vi "TemperatureControl_AVS.vi"(0 "T target":dbl, 5 "rate (K/min)":dbl=0.001, 9 "stop":bool, 11 "wait for T":bool, 12 "heater off":bool) -> (4 "T_set = T_target":bool)   [LabVIEW 2010]
uses:
  Instrument_Setup.vi
  Data_Display_global.vi
  Instance           1 36Saved   Temperaturkontrolle_Anfahren .vi
  Programme/National Instruments/LabVIEW 8.5/instr.lib/Mischerinstr.lib/AVS-Brücke/LV Drivers for AVS/AVS47IB.LLB/AVS47IB Wait for OPC/MAV/TMO.vi
  ControlCentre/Global 1.vi
panel:
  in  "Still value (mA)":dbl=0.7
  out "R":dbl=22.359058380126953 format="%.2f"
  out "activity":bool
  in  "excitation low T":dbl=4.0
  in  "change excitation":bool
  in  "excitation high T":dbl=4.0
  in  "from T (K)":dbl=0.15
  in  "?":bool
  in  "wait after sweep":u32
  in  "T max \nstill=on":dbl=0.7
  in  "still automatic":bool
  out "i=0":bool
  in  "change rate":bool
  in  "?":bool
  out "stability (K)":dbl
  in  "wait before start":u32=30
  in  "High-T mode":bool
  in  "from T (K)":dbl=0.5
  in  "change rate\nK/min":dbl=0.015
  in  "Delay (sec) 2":i16=1 min=0 max=3600 step=1
  out "T within\ntolerance":bool
  in  "stability \ntolerance (%)":dbl=1.0
  out "SetPoint":dbl
  out "T_set":dbl
  out "Delta t (sec)":dbl format="%.4f"
  in  "Delay (sec)":i16=1 min=0 max=3600 step=1
  out "T (K)":dbl=0.00957168277075326 format="%^.3e"
  in  "sweep tolerance %":dbl=0.1
  in  "critical temperature":dbl=0.8
  out "?":bool
  out "Down-Sweep":bool
  in  "tolerance T_set=T_target %":dbl=0.1
  out "resistance":dbl format="%.2f"
  out "T(K) history 2":dbl(graph)
  out "K  2":dbl format="%.4f"
  out "T(K) history3":dbl(graph)
  out "K":dbl format="%.4f"
  # "s"
  # "s"
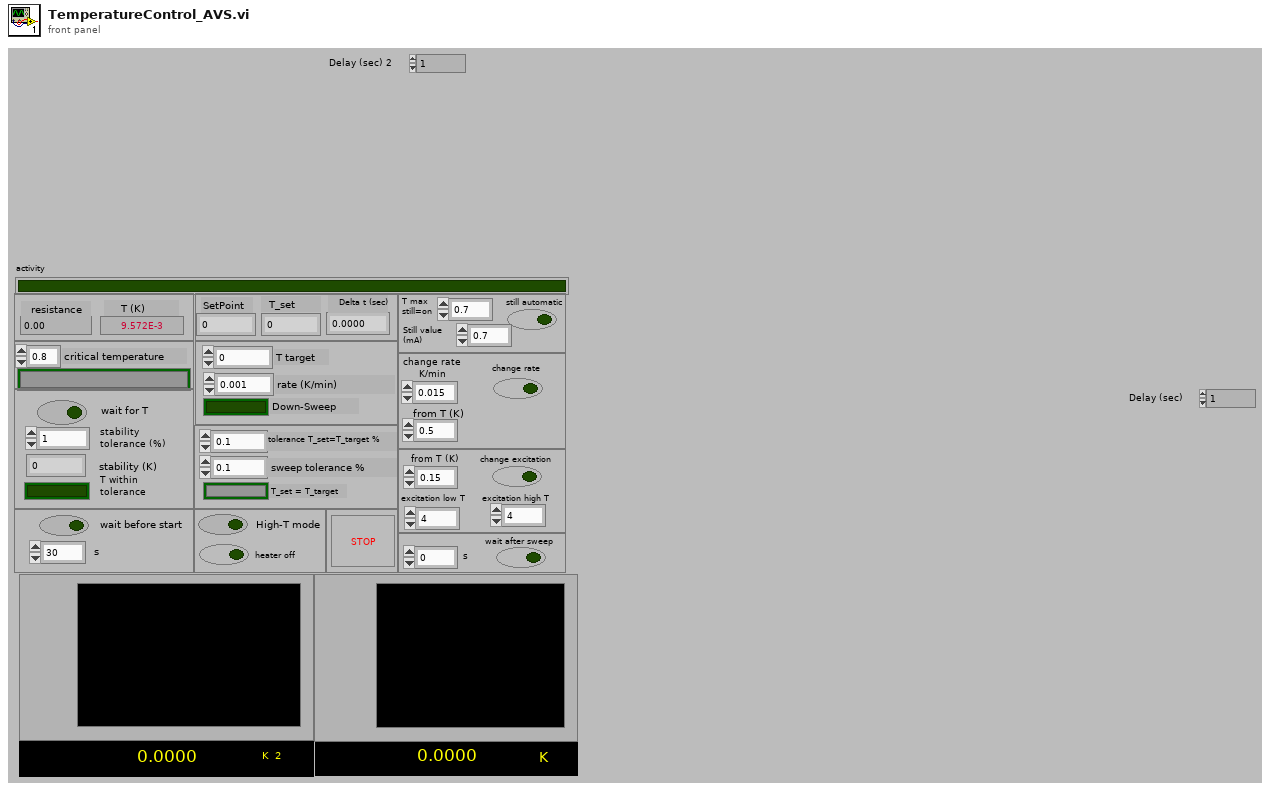
[diagram p1: front panel]
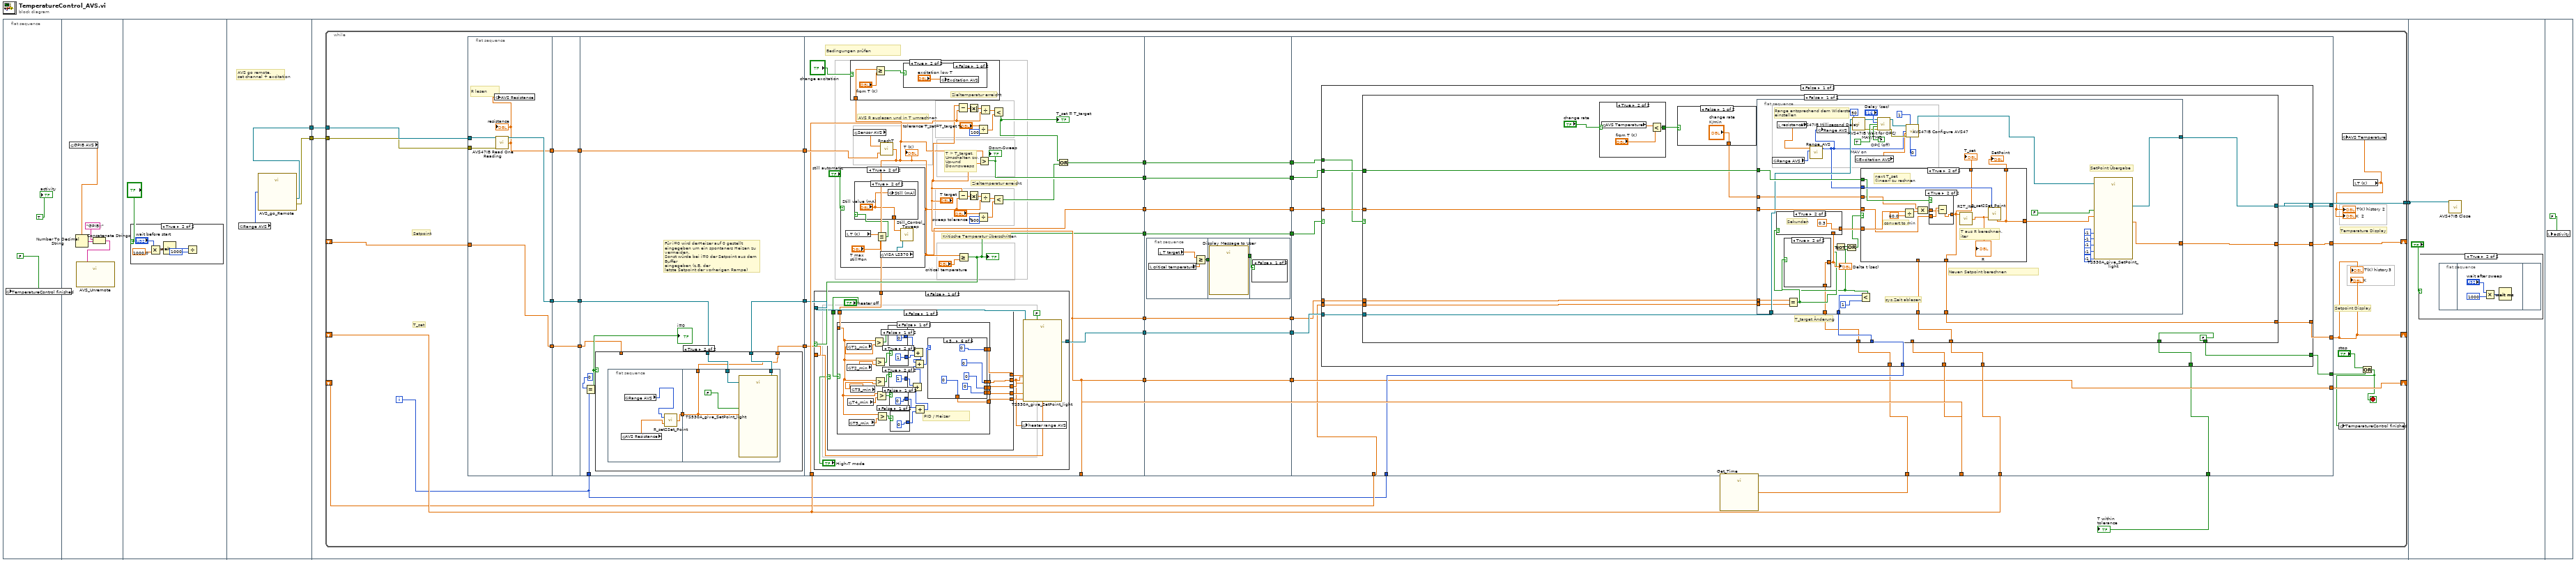
[diagram p0: block diagram]
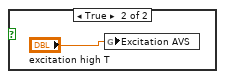
[diagram p5: hidden frame]
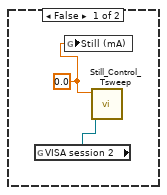
[diagram p6: hidden frame]
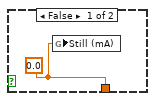
[diagram p7: hidden frame]
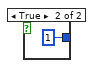
[diagram p8: hidden frame]
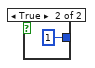
[diagram p9: hidden frame]
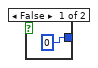
[diagram p10: hidden frame]
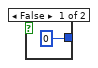
[diagram p11: hidden frame]
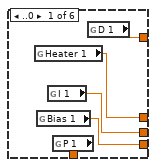
[diagram p12: hidden frame]
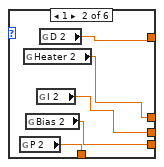
[diagram p13: hidden frame]
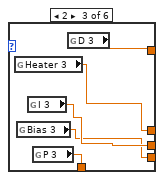
[diagram p14: hidden frame]
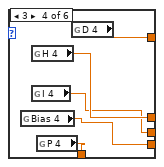
[diagram p15: hidden frame]
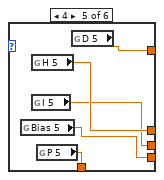
[diagram p16: hidden frame]
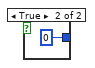
[diagram p17: hidden frame]
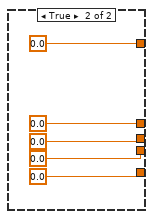
[diagram p18: hidden frame]
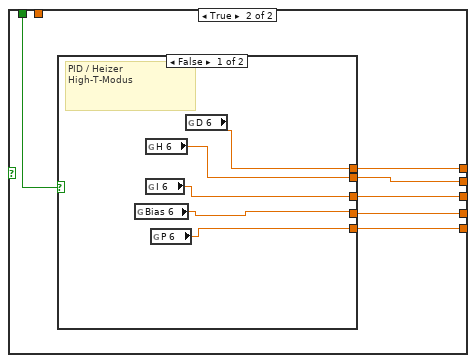
[diagram p19: hidden frame]
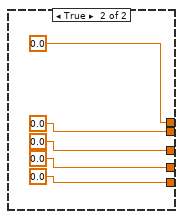
[diagram p20: hidden frame]
diagram:
  n1 = flat-sequence {
    tunnel: [w18] -> w3
    tunnel: [w17] -> w2
    tunnel: w3 -> [w21]
    tunnel: w2 -> [w20]
    tunnel: [w19] -> w1
    tunnel: w1 -> [w447]
    frame #0 {
      n2 = global write "Instrument_Setup.vi" "TemperatureControl finished"(FALSE) -> ()
      "activity" <- TRUE ("activity")
    }
    frame #1 {
      n3 = global read "Instrument_Setup.vi" "GPIB AVS"() -> (w6:dbl)
      n4 = Number To Decimal String(number=w6) -> (decimal integer string=w8:string)  [unwired: 1 in]
      n5 = Concatenate Strings("GPIB::", w8) -> (w7:string)
      n6 = call "AVS_Unremote.vi"("VISA session"=w7) -> ()  [unwired: 11 in]
    }
    frame #2 {
      n7 = case shown="True" "?" {
        frame False {
        }
        frame True {
          n8 = Multiply(x="wait before start", y=1000.0) -> (x*y=w13:dbl)
          n9 = Wait (ms)(milliseconds to wait=w13) -> (millisecond timer value=w12:u32)
          n10 = Divide(x=w12, y=u32 1000) -> ()  [unwired: 1 out]
        }
      }
    }
    frame #3 {
      # "AVS go remote,\nset channel + excitation"
      n11 = global read "Instrument_Setup.vi" "Range AVS"() -> (w16:i8)
      n12 = call "AVS_go_Remote.vi"("RANGE  (-1:no change)"=w16) -> ("error out"=w17:errorcluster, "dup VISA session"=w18:refnum<visa-resource-name>)
    }
    frame #4 {
      n13 = while {
        tunnel: w21 -> [w61]
        tunnel: w20 -> [w60]
        shift-right: [w59] -> _
        shift-left: _ -> [w58]
        shift-right: [w57] -> _
        shift-left: _ -> [w55]
        tunnel: [w56] -> w19
        shift-right: [w53] -> _
        shift-left: _ -> [w52]
        i -> [w46]
        stop <- w23 stop-if-true
        # "T_set"
        # "Setpoint"
        # "Setpoint Display"
        # "Temperature Display"
        n14 = flat-sequence {
          tunnel: [w62] -> w31
          tunnel: w61 -> [w66]
          tunnel: w60 -> [w65]
          tunnel: [w64] -> w29
          tunnel: [w63] -> w27
          tunnel: w55 -> [w63]
          tunnel: w31 -> [w69]
          tunnel: [w69] -> w30
          tunnel: w29 -> [w68]
          tunnel: [w68] -> w28
          tunnel: w27 -> [w67]
          tunnel: [w67] -> w26
          tunnel: w30 -> [w77]
          tunnel: [w77] -> w48
          tunnel: w28 -> [w73]
          tunnel: [w72] -> w47
          tunnel: w26 -> [w71]
          tunnel: w46 -> [w76]
          tunnel: [w70] -> w25
          tunnel: [w95] -> w45
          tunnel: w48 -> [w111]
          tunnel: [w91] -> w43
          tunnel: [w110] -> w41
          tunnel: w58 -> [w103]
          tunnel: w47 -> [w102]
          tunnel: [w101] -> w39
          tunnel: ["T target"] -> w54
          tunnel: ["T target"] -> w37
          tunnel: w25 -> [w98]
          tunnel: [w100] -> w35
          tunnel: ["T target"] -> w33
          tunnel: w45 -> [w247]
          tunnel: [w247] -> w44
          tunnel: w43 -> [w246]
          tunnel: [w246] -> w42
          tunnel: w41 -> [w245]
          tunnel: [w245] -> w40
          tunnel: w39 -> [w244]
          tunnel: [w244] -> w38
          tunnel: w37 -> [w243]
          tunnel: [w243] -> w36
          tunnel: w35 -> [w242]
          tunnel: [w242] -> w34
          tunnel: w33 -> [w241]
          tunnel: [w241] -> w32
          tunnel: w46 -> [w270]
          tunnel: [w269] -> w59
          tunnel: w44 -> [w268]
          tunnel: w58 -> [w267]
          tunnel: w42 -> [w266]
          tunnel: w40 -> [w265]
          tunnel: [w264] -> w57
          tunnel: [w263] -> w56
          tunnel: w38 -> [w262]
          tunnel: w36 -> [w261]
          tunnel: w34 -> [w260]
          tunnel: w54 -> [w259]
          tunnel: [w258] -> w53
          tunnel: w32 -> [w258]
          tunnel: w52 -> [w257]
          tunnel: [w256] -> w50
          tunnel: w49 -> [w255]
          tunnel: [w254] -> w24
          frame #0 {
            # "R lesen"
            n15 = call "AVS47IB Read One Reading.vi"("VISA session"=w66, "error in (no error)"=w65) -> ("dup VISA session"=w64:refnum<visa-resource-name>, "Resistance reading"=w62:dbl)  [unwired: 9 in, 3 out]
            "resistance" <- w62
            n16 = global write "Data_Display_global.vi" "AVS Resistance"(w62) -> ()
          }
          frame #1 {
          }
          frame #2 {
            # "Für i=0 wird derHeizer auf 0 gestellt\neingegeben um ein spontaners Heizen zu \nvermeiden.\nSonst würde bei i=0 der Setpoint aus dem Buffer\neingegeben (z.B. der \nletzte Setpoint der vorherigen Rampe)"
            n17 = Equal?(x=0, y=w76) -> (x = y?=w74:bool)
            "i=0" <- w74
            n18 = case shown="True" w74 {
              tunnel: w73 -> [w79 w83]
              tunnel: [w79 w82] -> w72
              tunnel: w71 -> [w78 _]
              tunnel: [w78 w80] -> w70
              frame False {
              }
              frame True {
                n19 = flat-sequence {
                  tunnel: [w86] -> w81
                  tunnel: w83 -> [w90]
                  tunnel: [w89] -> w82
                  tunnel: w81 -> [w87]
                  tunnel: [w87] -> w80
                  frame #0 {
                    n20 = global read "Data_Display_global.vi" "AVS Resistance"() -> (w84:dbl)
                    n21 = global read "Instrument_Setup.vi" "Range AVS"() -> (w85:i8)
                    n22 = call "R_set2Set_Point.vi"("range"=w85, "Widerstand_Target"=w84) -> ("SetPoint"=w86:dbl)  [unwired: 2 in]
                  }
                  frame #1 {
                    n23 = call "TS530A_give_SetPoint_light.vi"("Set Point"=w87, "dup VISA session"=w90, "ObAllein"=FALSE) -> ("dup VISA session 2"=w89:refnum<visa-resource-name>)  [unwired: 6 in, 1 out]
                  }
                }
              }
            }
          }
          frame #3 {
            # "T > T_target,\nUmschalten zw.\nUp-und \nDownsweeps"
            # "Kritische Temperatur überschritten"
            # "Zieltemperatur erreicht"
            # "Bedingungen prüfen"
            # "AVS R auslesen und in T umrechnen"
            n24 = case shown="True" "still automatic" {
              frame False {
                w124 = 0.0 ("Still (mA)")
                n25 = global read "Instrument_Setup.vi" "VISA session 2"() -> (w125:refnum<visa-resource-name>)
                n26 = global write "Instrument_Setup.vi" "Still (mA)"(w124) -> ()
                n27 = call "Still_Control_Tsweep.vi"("VISA session"=w125, "I (mA)"=w124) -> ()  [unwired: 10 in]
              }
              frame True {
                n28 = local read "T (K)"() -> (w129:dbl)
                n29 = Less Or Equal?(x=w129, y="T max \nstill=on") -> (x <= y?=w128:bool)
                n30 = case shown="True" w128 {
                  tunnel: [w131 "Still value (mA)"] -> w130
                  frame False {
                    w131 = 0.0 ("Still (mA)")
                    n31 = global write "Instrument_Setup.vi" "Still (mA)"(w131) -> ()
                  }
                  frame True {
                    n32 = global write "Instrument_Setup.vi" "Still (mA)"("Still value (mA)") -> ()
                  }
                }
                n33 = global read "Instrument_Setup.vi" "VISA LS370"() -> (w126:refnum<visa-resource-name>)
                n34 = call "Still_Control_Tsweep.vi"("VISA session"=w126, "I (mA)"=w130) -> ()  [unwired: 10 in]
              }
            }
            n35 = global read "Instrument_Setup.vi" "Sensor AVS"() -> (w92:dbl)
            n36 = call "RnachT.vi"("R"=w111, "Sensor Cal #"=w92) -> ("T (K)"=w91:dbl)
            "T (K)" <- w91
            n37 = case shown="True" "change excitation" {
              tunnel: w91 -> [_ w121]
              frame False {
              }
              frame True {
                # "Zieltemperatur erreicht"
                n38 = Greater Or Equal?(x=w121, y="from T (K)") -> (x >= y?=w119:bool)
                n39 = case shown="False" w119 {
                  frame False {
                    n40 = global write "Instrument_Setup.vi" "Excitation AVS"("excitation low T") -> ()
                  }
                  frame True {
                    n41 = global write "Instrument_Setup.vi" "Excitation AVS"("excitation high T") -> ()
                  }
                }
              }
            }
            n42 = Subtract(x="T target", y=w103) -> (x-y=w106:dbl)
            n43 = Subtract(x="T target", y=w91) -> (x-y=w114:dbl)
            n44 = Greater Or Equal?(x=w91, y="critical temperature") -> (x >= y?=w95:bool)
            "?" <- w95
            n45 = case shown="False" w95 {
              tunnel: w102 -> [w139 w238]
              tunnel: [w138 w238] -> w101
              tunnel: w98 -> [w137 _]
              tunnel: w91 -> [w136 _]
              frame False {
                n46 = case shown="False" "High-T mode" {
                  tunnel: [w151 w227] -> w144
                  tunnel: [w150 w226] -> w133
                  tunnel: [w149 w225] -> w143
                  tunnel: [w148 w224] -> w142
                  tunnel: [w147 w223] -> w141
                  tunnel: w136 -> [w146 _]
                  tunnel: "heater off" -> [w145 w222]
                  frame False {
                    n47 = case shown="False" w145 {
                      tunnel: [w170 0.0 ("D 5")] -> w151
                      tunnel: [w169 0.0 ("H 5")] -> w150
                      tunnel: [w168 0.0 ("I 5")] -> w149
                      tunnel: [w167 0.0 ("Bias 5")] -> w148
                      tunnel: [w166 0.0 ("P 5")] -> w147
                      tunnel: w146 -> [w157 _]
                      frame False {
                        # "PID / Heizer"
                        n48 = global read "Instrument_Setup.vi" "T1_min"() -> (w176:dbl)
                        n49 = global read "Instrument_Setup.vi" "T2_min"() -> (w175:dbl)
                        n50 = global read "Instrument_Setup.vi" "T4_min"() -> (w160:dbl)
                        n51 = global read "Instrument_Setup.vi" "T5_min"() -> (w158:dbl)
                        n52 = global read "Instrument_Setup.vi" "T3_min"() -> (w152:dbl)
                        n53 = Greater?(x=w157, y=w176) -> (0:w174:bool)
                        n54 = Greater?(x=w157, y=w175) -> (0:w173:bool)
                        n55 = Greater?(x=w157, y=w152) -> (0:w172:bool)
                        n56 = Greater?(x=w157, y=w160) -> (0:w159:bool)
                        n57 = Greater?(x=w157, y=w158) -> (0:w156:bool)
                        n58 = case shown="False" w174 {
                          tunnel: [0 0] -> w171
                          frame False {
                          }
                          frame True {
                          }
                        }
                        n59 = case shown="True" w172 {
                          tunnel: [0 1] -> w164
                          frame False {
                          }
                          frame True {
                          }
                        }
                        n60 = case shown="True" w173 {
                          tunnel: [0 1] -> w165
                          frame False {
                          }
                          frame True {
                          }
                        }
                        n61 = case shown="False" w159 {
                          tunnel: [0 1] -> w154
                          frame False {
                          }
                          frame True {
                          }
                        }
                        n62 = case shown="False" w156 {
                          tunnel: [0 1] -> w155
                          frame False {
                          }
                          frame True {
                          }
                        }
                        n63 = Add(x=w171, y=w165) -> (x+y=w162:i32)
                        n64 = Add(x=w154, y=w155) -> (x+y=w153:i32)
                        n65 = Add(x=w164, y=w153) -> (x+y=w161:i32)
                        n66 = Add(x=w162, y=w161) -> (x+y=w163:i32)
                        n67 = case shown="5.." w163 {
                          tunnel: [w189 w194 w199 w204 w209 0] -> w170
                          tunnel: [w185 w193 w198 w203 w208 0] -> w169
                          tunnel: [w188 w192 w197 w202 w207 0] -> w168
                          tunnel: [w187 w191 w196 w201 w206 0] -> w167
                          tunnel: [w186 w190 w195 w200 w205 0] -> w166
                          frame ..0 {
                            n68 = global read "Instrument_Setup.vi" "Heater 1"() -> (w185:dbl)
                            n69 = global read "Instrument_Setup.vi" "Bias 1"() -> (w187:dbl)
                            n70 = global read "Instrument_Setup.vi" "I 1"() -> (w188:dbl)
                            n71 = global read "Instrument_Setup.vi" "P 1"() -> (w186:dbl)
                            n72 = global read "Instrument_Setup.vi" "D 1"() -> (w189:dbl)
                          }
                          frame 1 {
                            n73 = global read "Instrument_Setup.vi" "P 2"() -> (w190:dbl)
                            n74 = global read "Instrument_Setup.vi" "Heater 2"() -> (w193:dbl)
                            n75 = global read "Instrument_Setup.vi" "Bias 2"() -> (w191:dbl)
                            n76 = global read "Instrument_Setup.vi" "I 2"() -> (w192:dbl)
                            n77 = global read "Instrument_Setup.vi" "D 2"() -> (w194:dbl)
                          }
                          frame 2 {
                            n78 = global read "Instrument_Setup.vi" "Heater 3"() -> (w198:dbl)
                            n79 = global read "Instrument_Setup.vi" "Bias 3"() -> (w196:dbl)
                            n80 = global read "Instrument_Setup.vi" "I 3"() -> (w197:dbl)
                            n81 = global read "Instrument_Setup.vi" "P 3"() -> (w195:dbl)
                            n82 = global read "Instrument_Setup.vi" "D 3"() -> (w199:dbl)
                          }
                          frame 3 {
                            n83 = global read "Instrument_Setup.vi" "Bias 4"() -> (w201:dbl)
                            n84 = global read "Instrument_Setup.vi" "H 4"() -> (w203:dbl)
                            n85 = global read "Instrument_Setup.vi" "I 4"() -> (w202:dbl)
                            n86 = global read "Instrument_Setup.vi" "P 4"() -> (w200:dbl)
                            n87 = global read "Instrument_Setup.vi" "D 4"() -> (w204:dbl)
                          }
                          frame 4 {
                            n88 = global read "Instrument_Setup.vi" "Bias 5"() -> (w206:dbl)
                            n89 = global read "Instrument_Setup.vi" "H 5"() -> (w208:dbl)
                            n90 = global read "Instrument_Setup.vi" "I 5"() -> (w207:dbl)
                            n91 = global read "Instrument_Setup.vi" "P 5"() -> (w205:dbl)
                            n92 = global read "Instrument_Setup.vi" "D 5"() -> (w209:dbl)
                          }
                          frame 5.. {
                          }
                        }
                      }
                      frame True {
                      }
                    }
                  }
                  frame True {
                    n93 = case shown="False" w222 {
                      tunnel: [w232 0.0 ("D 5")] -> w227
                      tunnel: [w231 0.0 ("H 5")] -> w226
                      tunnel: [w230 0.0 ("I 5")] -> w225
                      tunnel: [w229 0.0 ("Bias 5")] -> w224
                      tunnel: [w228 0.0 ("P 5")] -> w223
                      frame False {
                        # "PID / Heizer\nHigh-T-Modus"
                        n94 = global read "Instrument_Setup.vi" "Bias 6"() -> (w229:dbl)
                        n95 = global read "Instrument_Setup.vi" "H 6"() -> (w231:dbl)
                        n96 = global read "Instrument_Setup.vi" "I 6"() -> (w230:dbl)
                        n97 = global read "Instrument_Setup.vi" "P 6"() -> (w228:dbl)
                        n98 = global read "Instrument_Setup.vi" "D 6"() -> (w232:dbl)
                      }
                      frame True {
                      }
                    }
                  }
                }
                n99 = global write "Instrument_Setup.vi" "heater range AVS"(w133) -> ()
                n100 = call "TS530A_give_SetPoint_light.vi"("Set Point"=w137, "dup VISA session"=w139, "ObAllein"=FALSE, "PROPORTIONAL GAIN"=w141, "INTEGRATOR TC"=w143, "DERIVATOR TC"=w144, "HEATER POWER RANGE"=w133, "POWER BIAS"=w142) -> ("dup VISA session 2"=w138:refnum<visa-resource-name>)  [unwired: 1 in, 1 out]
              }
              frame True {
              }
            }
            n101 = Absolute Value(x=w106) -> (abs(x)=w107:dbl)
            n102 = Absolute Value(x=w114) -> (abs(x)=w115:dbl)
            n103 = Divide(x="tolerance T_set=T_target %", y=100) -> (x/y=w109:dbl)
            n104 = Divide(x="sweep tolerance %", y=100) -> (x/y=w117:dbl)
            n105 = Greater?(x=w91, y="T target") -> (0:w110:bool)
            "Down-Sweep" <- w110
            n106 = Divide(x=w107, y=w103) -> (x/y=w108:dbl)
            n107 = Divide(x=w115, y=w91) -> (x/y=w116:dbl)
            n108 = Less?(x=w108, y=w109) -> (x < y?=w99:bool)
            "T_set = T_target" <- w99
            n109 = Less?(x=w116, y=w117) -> (x < y?=w96:bool)
            n110 = Or(x=w99, y=w96) -> (x .or. y?=w100:bool)
          }
          frame #4 {
            n111 = flat-sequence {
              tunnel: [w248] -> w240
              tunnel: w240 -> [w251]
              tunnel: [w251] -> w239
              tunnel: w239 -> [w252]
              frame #0 {
                n112 = local read "critical temperature"() -> (w249:dbl)
                n113 = local read "T target"() -> (w250:dbl)
                n114 = Greater Or Equal?(x=w250, y=w249) -> (x >= y?=w248:bool)
              }
              frame #1 {
                n115 = call "Display Message to User"("Enable"=w251) -> ()  [unwired: 9 in, 2 out]
              }
              frame #2 {
                n116 = case shown="False" w252 {
                  frame False {
                  }
                  frame True {
                    n117 = Wait (ms)(milliseconds to wait=u32 10000) -> ()  [unwired: 1 out]
                  }
                }
              }
            }
          }
          frame #5 {
            n118 = case shown="False" w268 {
              tunnel: w270 -> [w285 _]
              tunnel: [w284 w444] -> w269
              tunnel: w267 -> [w283 w444]
              tunnel: w266 -> [w282 _]
              tunnel: w265 -> [w281 _]
              tunnel: [w280 w443] -> w264
              tunnel: [w279 w441] -> w263
              tunnel: w262 -> [w278 w442]
              tunnel: w261 -> [w277 _]
              tunnel: w260 -> [w274 _]
              tunnel: w259 -> [w276 _]
              tunnel: w257 -> [w275 _]
              tunnel: [w273 w440] -> w256
              tunnel: w255 -> [w272 _]
              tunnel: [w271 w440] -> w254
              frame False {
                n119 = case shown="False" w274 {
                  tunnel: w285 -> [w300 _]
                  tunnel: [w299 w394] -> w284
                  tunnel: w283 -> [w298 _]
                  tunnel: w282 -> [w297 _]
                  tunnel: w281 -> [w296 _]
                  tunnel: [w295 w395] -> w280
                  tunnel: [w294 w396] -> w279
                  tunnel: w278 -> [w293 w397]
                  tunnel: w277 -> [w292 _]
                  tunnel: w276 -> [_ w394]
                  tunnel: w275 -> [w291 _]
                  tunnel: [w289 w391] -> w273
                  tunnel: w272 -> [w290 _]
                  tunnel: [w289 w389] -> w271
                  frame False {
                    w289 = FALSE ("T innerhalb Toleranz")
                    # "T_target Änderung"
                    n120 = case shown="True" "change rate" {
                      tunnel: [TRUE w304] -> w288
                      frame False {
                      }
                      frame True {
                        n121 = global read "Data_Display_global.vi" "AVS Temperature"() -> (w302:dbl)
                        n122 = Less?(x=w302, y="from T (K)") -> (x < y?=w304:bool)
                      }
                    }
                    n123 = case shown="False" w288 {
                      tunnel: ["change rate\nK/min" "rate (K/min)"] -> w287
                      frame False {
                      }
                      frame True {
                      }
                    }
                    n124 = flat-sequence {
                      tunnel: w300 -> [w318]
                      tunnel: [w346] -> w299
                      tunnel: w298 -> [w345]
                      tunnel: w297 -> [w339]
                      tunnel: w296 -> [w335]
                      tunnel: [w334] -> w295
                      tunnel: [w323] -> w294
                      tunnel: w293 -> [w325]
                      tunnel: w292 -> [w322]
                      tunnel: w291 -> [w315]
                      tunnel: w290 -> [w314]
                      tunnel: w287 -> [w312]
                      frame #0 {
                        w332 = FALSE  # OPC (off)
                        w333 = TRUE  # MAV on
                        # "sys.Zeit ablesen"
                        # "Range entsprechend dem Widerstand\neinstellen"
                        # "SetPoint Übergabe"
                        # "Neuen Setpoint berechnen"
                        n125 = global read "Instrument_Setup.vi" "Range AVS"() -> (w309:i8)
                        n126 = local read "resistance"() -> (w308:dbl)
                        n127 = Equal?(x=w322, y=w315) -> (x = y?=w319:bool)
                        n128 = case shown="True" w319 {
                          tunnel: [0.3 ("Delta t (sec)") w351] -> w336
                          tunnel: w314 -> [_ w351]
                          frame False {
                          }
                          frame True {
                          }
                        }
                        "Delta t (sec)" <- w336
                        n129 = call "Range_AVS.vi"("old range"=w309, "Widerstand"=w308) -> ("new range"=w307:i8)  [unwired: 9 in]
                        n130 = global write "Instrument_Setup.vi" "Range AVS"(w307) -> ()
                        n131 = Not(x=w319) -> (.not. x?=w320:bool)
                        n132 = call "AVS47IB Millisecond Delay.vi"("VISA session"=w325, "Delay (50 ms)"=50) -> ("dup VISA session"=w330:refnum<visa-resource-name>, "error out"=w329:errorcluster)  [unwired: 12 in]
                        n133 = global read "Instrument_Setup.vi" "Excitation AVS"() -> (w310:dbl)
                        n134 = Less?(x=w318, y=1 ("x")) -> (x < y?=w316:bool)
                        n135 = case shown="True" w316 {
                          tunnel: [w352 0.3 ("Delta t (sec)")] -> w349
                          tunnel: w336 -> [w352 _]
                          frame False {
                          }
                          frame True {
                            # "Sekunden"
                          }
                        }
                        n136 = Or(x=w320, y=w316) -> (x .or. y?=w321:bool)
                        n137 = case shown="True" w321 {
                          tunnel: w349 -> [w364 w379]
                          tunnel: [w356 w373] -> w348
                          tunnel: [w357 w374] -> w346
                          tunnel: w345 -> [w359 _]
                          tunnel: w307 -> [w358 w376]
                          tunnel: w339 -> [_ w375]
                          tunnel: [w357 w374] -> w338
                          tunnel: [w356 w373] -> w337
                          tunnel: w335 -> [w355 w372]
                          tunnel: w312 -> [w354 w371]
                          frame False {
                            # "next T_set \n(linear) zu rechnen"
                            # "convert to min"
                            n138 = Divide(x=w364, y=60.0) -> (x/y=w362:dbl)
                            n139 = Compound Arithmetic op=MULTIPLY(w354, w362) -> (w361:dbl)
                            n140 = case shown="True" w355 {
                              tunnel: w361 -> [w367 w368]
                              tunnel: w359 -> [w366 w369]
                              tunnel: [w365 w370] -> w357
                              frame False {
                                n141 = Add(x=w367, y=w366) -> (x+y=w365:dbl)
                              }
                              frame True {
                                n142 = Subtract(x=w369, y=w368) -> (x-y=w370:dbl)
                              }
                            }
                            n143 = call "R2T_Iter.vi"("T-Ziel"=w357) -> ("R"=w360:dbl)  [unwired: 1 in]
                            n144 = call "R_set2Set_Point.vi"("range"=w358, "Widerstand_Target"=w360) -> ("SetPoint"=w356:dbl)  [unwired: 2 in]
                          }
                          frame True {
                            # "T aus R berechnen,\niter"
                            # "next T_set \n(linear) zu rechnen"
                            # "convert to min"
                            n145 = Divide(x=w379, y=60.0) -> (x/y=w377:dbl)
                            n146 = Compound Arithmetic op=MULTIPLY(w371, w377) -> (w381:dbl)
                            n147 = case shown="True" w372 {
                              tunnel: w381 -> [w384 w385]
                              tunnel: w375 -> [w383 w386]
                              tunnel: [w382 w387] -> w374
                              frame False {
                                n148 = Add(x=w384, y=w383) -> (x+y=w382:dbl)
                              }
                              frame True {
                                n149 = Subtract(x=w386, y=w385) -> (x-y=w387:dbl)
                              }
                            }
                            n150 = call "R2T_Iter.vi"("T-Ziel"=w374) -> ("R"=w378:dbl)  [unwired: 1 in]
                            "R" <- w378
                            n151 = call "R_set2Set_Point.vi"("range"=w376, "Widerstand_Target"=w378) -> ("SetPoint"=w373:dbl)  [unwired: 2 in]
                          }
                        }
                        "SetPoint" <- w337
                        "T_set" <- w338
                        n152 = call "AVS47IB Wait for OPC/MAV/TMO.vi"("VISA session"=w330, "Timeout (2 sec)"="Delay (sec)", "MAV (on)"=w333, "OPC (off)"=w332, "error in (no error)"=w329) -> ("dup VISA session"=w327:refnum<visa-resource-name>, "error out"=w326:errorcluster)  [unwired: 8 in, 1 out]
                        n153 = call "AVS47IB Configure AVS47.vi"("VISA session"=w327, "INPUT (-1:no change)"=i8 1, "RANGE  (-1:no change)"=w307, "EXCITATION (-1:no change)"=w310, "error in (no error)"=w326, "DISPLAY (-1:no change)"=i8 0) -> ("dup VISA session"=w324:refnum<visa-resource-name>)  [unwired: 8 in, 1 out]
                        n154 = call "TS530A_give_SetPoint_light.vi"("Set Point"=w348, "dup VISA session"=w324, "ObAllein"=FALSE, "PROPORTIONAL GAIN"=i8 -1, "INTEGRATOR TC"=i8 -1, "DERIVATOR TC"=i8 -1, "HEATER POWER RANGE"=i8 -1, "POWER BIAS"=i8 -1) -> ("set point"=w334:dbl, "dup VISA session 2"=w323:refnum<visa-resource-name>)  [unwired: 1 in]
                      }
                    }
                  }
                  frame True {
                    n155 = flat-sequence {
                      tunnel: w397 -> [w406]
                      tunnel: [w418] -> w393
                      tunnel: [w417] -> w392
                      tunnel: [w404] -> w390
                      tunnel: [w404] -> w388
                      tunnel: [w428] -> w395
                      tunnel: [w426] -> w396
                      tunnel: w393 -> [w427]
                      tunnel: w392 -> [w428]
                      tunnel: [w425] -> w391
                      tunnel: w390 -> [w424]
                      tunnel: [w423] -> w389
                      tunnel: w388 -> [w422]
                      frame #0 {
                        w414 = FALSE  # OPC (off)
                        w415 = TRUE  # MAV on
                        # "Range entsprechend dem Widerstand\neinstellen"
                        # "Wenn Zieltemperatur erreicht ist, gibt das Programm\nden zugehörigen Setpoint an die TS weiter und bleibt\ndann in einer Endlosschleife,\ndie durch einen Stopbefehl beendet werden kann."
                        n156 = global read "Instrument_Setup.vi" "Range AVS"() -> (w399:i8)
                        n157 = local read "resistance"() -> (w400:dbl)
                        n158 = call "Range_AVS.vi"("old range"=w399, "Widerstand"=w400) -> ("new range"=w398:i8)  [unwired: 9 in]
                        n159 = global write "Instrument_Setup.vi" "Range AVS"(w398) -> ()
                        n160 = call "AVS47IB Millisecond Delay.vi"("VISA session"=w406, "Delay (50 ms)"=50) -> ("dup VISA session"=w412:refnum<visa-resource-name>, "error out"=w411:errorcluster)  [unwired: 12 in]
                        n161 = global read "Instrument_Setup.vi" "Excitation AVS"() -> (w401:dbl)
                        n162 = call "AVS47IB Wait for OPC/MAV/TMO.vi"("VISA session"=w412, "Timeout (2 sec)"="Delay (sec) 2", "MAV (on)"=w415, "OPC (off)"=w414, "error in (no error)"=w411) -> ("dup VISA session"=w409:refnum<visa-resource-name>, "error out"=w408:errorcluster)  [unwired: 8 in, 1 out]
                        n163 = call "AVS47IB Configure AVS47.vi"("VISA session"=w409, "INPUT (-1:no change)"=i8 1, "RANGE  (-1:no change)"=w398, "EXCITATION (-1:no change)"=w401, "error in (no error)"=w408, "DISPLAY (-1:no change)"=i8 0) -> ("dup VISA session"=w405:refnum<visa-resource-name>)  [unwired: 8 in, 1 out]
                        n164 = local read "T target"() -> (w404:dbl)
                        n165 = call "R2T_Iter.vi"("T-Ziel"=w404) -> ("R"=w416:dbl)  [unwired: 1 in]
                        n166 = global read "Instrument_Setup.vi" "Range AVS"() -> (w402:i8)
                        n167 = call "R_set2Set_Point.vi"("range"=w402, "Widerstand_Target"=w416) -> ("SetPoint"=w420:dbl)  [unwired: 2 in]
                        n168 = Wait (ms)(milliseconds to wait=u32 500) -> ()  [unwired: 1 out]
                        n169 = call "TS530A_give_SetPoint_light.vi"("Set Point"=w420, "dup VISA session"=w405) -> ("set point"=w417:dbl, "dup VISA session 2"=w418:refnum<visa-resource-name>)  [unwired: 7 in]
                      }
                      frame #1 {
                        n170 = case shown="False" "wait for T" {
                          tunnel: w427 -> [w430 w439]
                          tunnel: [w430 w438] -> w426
                          tunnel: [w429 w431] -> w425
                          tunnel: w424 -> [_ w437]
                          tunnel: [w429 w431] -> w423
                          tunnel: w422 -> [_ w436]
                          frame False {
                            w429 = TRUE ("T innerhalb Toleranz")
                          }
                          frame True {
                            n171 = Divide(x=w436, y=100.0) -> (x/y=w433:dbl)
                            n172 = Multiply(x="stability \ntolerance (%)", y=w433) -> (x*y=→"stability (K)":dbl)
                            n173 = call "wait_for_T_v2.vi"("Toleranz (%)"="stability \ntolerance (%)", "VISA session 2"=w439, "T_target"=w437) -> ("dup VISA session"=w438:refnum<visa-resource-name>, "T innerhalb Toleranz"=w431:bool)  [unwired: 7 in]
                          }
                        }
                      }
                    }
                  }
                }
              }
              frame True {
                w440 = FALSE
                # "Heizer aus"
                n174 = global read "Global 1.vi" "GPIB TS"() -> (w445:dbl)
                n175 = call "TS530A_give_SetPoint_light.vi"("Set Point"=w445, "dup VISA session"=w442, "HEATER POWER RANGE"=i8 0) -> ("set point"=w443:dbl, "dup VISA session 2"=w441:refnum<visa-resource-name>)  [unwired: 6 in]
              }
            }
          }
        }
        n176 = call "Get_Time.vi"() -> ("Delta t (sec)"=w49:dbl)  [unwired: 2 out]
        n177 = local read "T (K)"() -> (w22:dbl)
        "T(K) history 2" <- w22
        "K  2" <- w22
        n178 = global write "Data_Display_global.vi" "AVS Temperature"(w22) -> ()
        n179 = Or(x="stop", y=w50) -> (x .or. y?=w23:bool)
        n180 = global write "Instrument_Setup.vi" "TemperatureControl finished"(w23) -> ()
        "T(K) history3" <- w59
        "K" <- w59
        "T within\ntolerance" <- w24
      }
    }
    frame #5 {
      n181 = case shown="True" "?" {
        frame False {
        }
        frame True {
          n182 = flat-sequence {
            frame #0 {
            }
            frame #1 {
              n183 = Multiply(x="wait after sweep", y=u32 1000) -> (x*y=w450:u32)
              n184 = Wait (ms)(milliseconds to wait=w450) -> ()  [unwired: 1 out]
            }
            frame #2 {
            }
          }
        }
      }
      n185 = call "AVS47IB Close.vi"("VISA session"=w447) -> ()  [unwired: 14 in, 1 out]
    }
    frame #6 {
      n186 = local write "activity"(FALSE ("activity")) -> ()
    }
  }
